vi "Install All.vi"(7 "Restart Automatically (T)":bool=TRUE, 8 "error in (no error)":errorcluster, 10 "Deselect Conflicts (F)":bool, 11 "Session in":refnum<k21>) -> (0 "error out":errorcluster, 1 "Broken Dependencies":T1[](array[typedef]) {"dependee"."component type" items=["standard", "hidden", "system", "unknown", "startup", "image", "essential"]; "depender"."component type" items=["standard", "hidden", "system", "unknown", "startup", "image", "essential"]}, 2 "Installed Software":T2[](array[typedef]) {"component type" items=["standard", "hidden", "system", "unknown", "startup", "image", "essential"]}, 3 "Session out":refnum<k21>)   [LabVIEW 2020, in "nisyscfg.lvlib"]
doc: "Use the Install All VI to install the highest installable version of all available components, even if the component(s) are already installed on the target."
uses:
  <vilib>/nisyscfg/nisyscfg.lvlib
  <vilib>/nisyscfg/Software 1.2.ctl
  <vilib>/nisyscfg/Component Type.ctl
  <vilib>/nisyscfg/Broken Dependency 1.2.ctl
  <vilib>/Utility/error.llb/Error Cluster From Error Code.vi
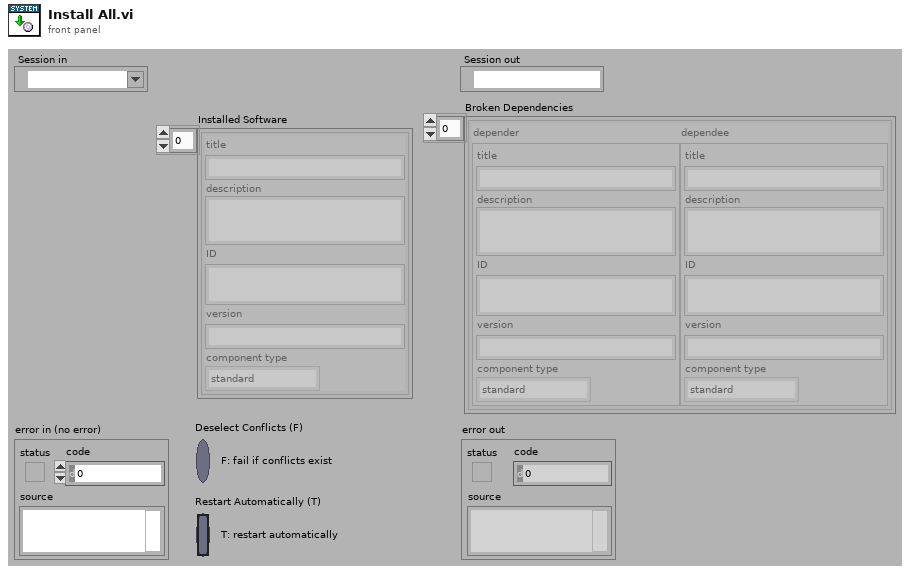
[diagram p1: front panel]
types:
  T1 = typedef "nisyscfg.lvlib/Broken Dependency 1.2.ctl" = cluster{"depender":T2, "dependee":T2}
  T2 = typedef "nisyscfg.lvlib/Software 1.2.ctl" = cluster{"title":string, "description":string, "ID":string, "version":string, "component type":T3}
  T3 = typedef "nisyscfg.lvlib/Component Type.ctl" = u32
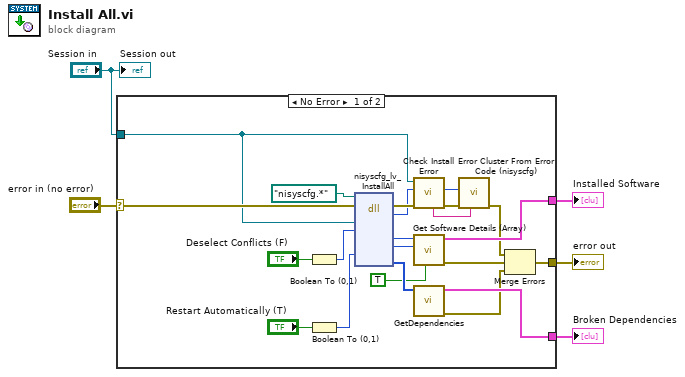
[diagram p0: block diagram]
diagram:
  n1 = case shown="No Error" "error in (no error)" {
    selector: "error in (no error)" -> [w16 w28]
    tunnel: [w21 _] -> w5
    tunnel: [w13 w28] -> w4
    tunnel: "Session in" -> [w11 _]
    tunnel: [w24 _] -> w3
    frame No Error {
      n2 = Boolean To (0,1)(Boolean="Deselect Conflicts (F)") -> (0, 1=w26:i16)
      n3 = Boolean To (0,1)(Boolean="Restart Automatically (T)") -> (0, 1=w14:i16)
      n4 = dll-call lib="nisyscfg.*" fn="nisyscfg_lv_InstallAll" label="InstallAll"(path in=path "nisyscfg.*", error in=w16, "system"=w11, "deselectConflicts"=w26, "restartAutomatically"=w14) -> (error out=w10:errorcluster, "result"=w9:i32, "softwareNoConflicts"=w22:u64, "numSoftwareNoConflicts"=w18:i32, "brokenDependencies"=w25:u64[])  [unwired: 7 in, 1 out]
      n5 = call <vilib>:"Check Install Error.vi"("error in (no error)"=w10, "Status in"=w9, "Session in"=w11) -> ("error out"=w12:errorcluster, "Status out"=w7:i32, "Details"=w6:string)  [unwired: 5 in, 1 out]
      n6 = call <vilib>:"Get Software Details (Array).vi"("Trace Component Info (F)"=TRUE ("log to NI Spy (F)"), "Number of Elements"=w18, "Enumerator in"=w22) -> ("error out"=w20:errorcluster, "Software Components"=w21:T2[])  [unwired: 7 in]
      n7 = call <vilib>:"GetDependencies.vi"("Enumerator in"=w25) -> ("error out"=w19:errorcluster, "Dependencies"=w24:T1[])  [unwired: 9 in]
      n8 = call <vilib>:"Error Cluster From Error Code (nisyscfg).vi"("Details String"=w6, "error in (no error)"=w12, "Error Code (0)"=w7) -> ("error out"=w8:errorcluster)  [unwired: 8 in]
      n9 = Merge Errors(w8, w20, w19) -> (w13:errorcluster)
    }
    frame Error {
    }
  }
  "error out" <- w4
  "Installed Software" <- w5
  "Broken Dependencies" <- w3
  "Session out" <- "Session in"
